vi "Config - Update Data.vi"(8 "error in (no error)":errorcluster, 10 "Data Record":T1) -> (0 "error out":errorcluster)   [LabVIEW 2017]
doc: "Updates configuration data record into external XML file."
uses:
  Controls/Config Data Record.ctl
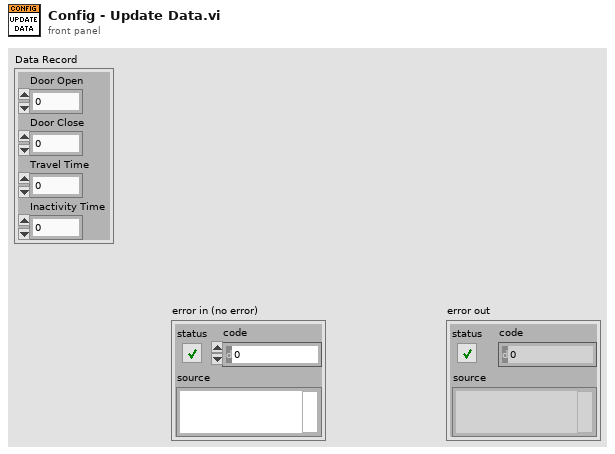
[diagram p1: front panel]
types:
  T1 = typedef "Config Data Record.ctl" = cluster{"Door Open":dbl, "Door Close":dbl, "Travel Time":dbl, "Inactivity Time":dbl}
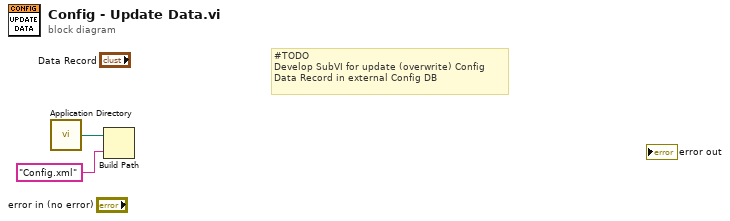
[diagram p0: block diagram]
diagram:
  # "#TODO\nDevelop SubVI for update (overwrite) Config\nData Record in external Config DB"
  n1 = call <vilib>:"Application Directory.vi"() -> ("Application Directory"=w2:path)
  n2 = Build Path(base path=w2, name or relative path="Config.xml") -> ()  [unwired: 1 out]
